vi "CS POLARIS BME DG Client.contents.vi"   [LabVIEW 2009, in "CS POLARIS BME DG Client.lvlib"]
uses:
  CS POLARIS BME DG Client.lvlib
types:
  T1 = typedef "CS POLARIS BME DG Client.lvlib/CS POLARIS BME DG Client.i attribute.ctl" = cluster{"Delay Formula Ref":refnum<vi>, "Active Ref":refnum<vi>, "OutputModulo Ref":refnum<vi>, "Rep Rate Ref":refnum<vi>, "Next Shot Ref":refnum<vi>, "Error Ref":refnum<vi>, "Switch Ref":refnum<vi>, "New Delay Formula Ref":refnum<vi>, "New OutputModulo Ref ":refnum<vi>, "Channel":string, "CS DG Obj":string, "Stop Ref":refnum<vi>, "Max delay change":dbl, "Enabled fields":u8, "LockInfo Ref":refnum<vi>}
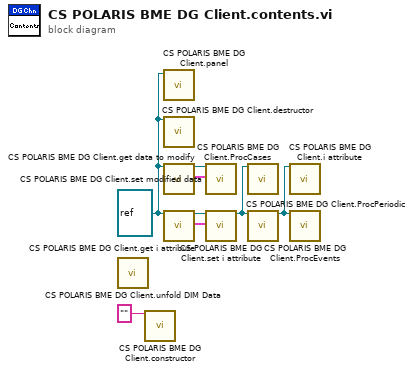
[diagram p0: block diagram]
diagram:
  w5 = refnum<vi> refnum ("object ref")
  n1 = call "CS POLARIS BME DG Client.unfold DIM Data.vi"() -> ()  [unwired: 13 in, 7 out]
  n2 = call "CS POLARIS BME DG Client.constructor.vi"("name"="") -> ()  [unwired: 16 in, 3 out]
  n3 = call "CS POLARIS BME DG Client.panel.vi"("object ref"=w5) -> ()  [unwired: 10 in, 1 out]
  n4 = call "CS POLARIS BME DG Client.destructor.vi"("i ref in"=w5) -> ()  [unwired: 18 in, 1 out]
  n5 = call "CS POLARIS BME DG Client.get data to modify.vi"("i ref in"=w5) -> ("i ref out"=w8:refnum<vi>, "i attribute"=w7:T1)  [unwired: 15 in, 2 out]
  n6 = call "CS POLARIS BME DG Client.get i attribute.vi"("i ref in"=w5) -> ("i ref out"=w4:refnum<vi>, "i attribute"=w3:T1)  [unwired: 16 in, 1 out]
  n7 = call "CS POLARIS BME DG Client.set modified data.vi"("i ref in"=w8, "i attribute"=w7) -> ()  [unwired: 16 in, 2 out]
  n8 = call "CS POLARIS BME DG Client.set i attribute.vi"("i ref in"=w4, "i attribute"=w3) -> ("i ref out"=w2:refnum<vi>)  [unwired: 16 in, 1 out]
  n9 = call "CS POLARIS BME DG Client.ProcCases.vi"("i ref in"=w2) -> ()  [unwired: 16 in, 3 out]
  n10 = call "CS POLARIS BME DG Client.ProcPeriodic.vi"("i ref in"=w2) -> ("i ref out"=w1:refnum<vi>)  [unwired: 16 in, 2 out]
  n11 = call "CS POLARIS BME DG Client.i attribute.vi"("VI Refnum"=w1) -> ()  [unwired: 16 in, 3 out]
  n12 = call "CS POLARIS BME DG Client.ProcEvents.vi"("i ref in"=w1) -> ()  [unwired: 17 in, 2 out]
